vi "capstone2 ver 1.vi"() -> ()   [LabVIEW 2016]
uses:
  <instrlib>/Dynamixel Motor/Public/Motor Operation/Low Level/Baud Setting.ctl
  <vilib>/myRIO/Instrument Drivers/Onboard IO/DIO/typedefs/DIO Reference.ctl
  <vilib>/myRIO/Common/Instrument Driver Framework/Utilities/typedefs/myRIO Generic Hardware Reference.ctl
  <vilib>/myRIO/Common/Instrument Driver Framework/Utilities/typedefs/Hardware Version Enum.ctl
  <vilib>/myRIO/Common/Instrument Driver Framework/Utilities/typedefs/myRIO v1.0 Reference.ctl
  <vilib>/myRIO/Common/Instrument Driver Framework/Utilities/typedefs/Generic FPGA Reference.ctl
  <vilib>/myRIO/Common/Instrument Driver Framework/myRIO v1.0/DIO/typedefs/DIO Channels List.ctl
  <vilib>/myRIO/Common/Instrument Driver Framework/myRIO v1.0/DIO/typedefs/DIO Channels Enum.ctl
  <vilib>/userdefined/High Color/nirio_resource_hc.ctl
  <vilib>/myRIO/Common/Instrument Driver Framework/Utilities/vis/Is FPGA Ref Available.vi
  <vilib>/myRIO/Common/Instrument Driver Framework/myRIO v1.0/DIO/vis/myRIO v1.1 Open DIO.vi
  <vilib>/myRIO/Instrument Drivers/Onboard IO/DIO/vis/Write.vi
  <vilib>/myRIO/Common/Instrument Driver Framework/Utilities/vis/Validate Channels.vi
  <vilib>/myRIO/Common/Instrument Driver Framework/myRIO v1.0/DIO/vis/myRIO v1.0 Reserve DIO.vi
  <vilib>/myRIO/Common/Instrument Driver Framework/myRIO v1.0/UART/vis/myRIO v1.0 Close UART.vi
  <vilib>/myRIO/Common/Instrument Driver Framework/myRIO v1.0/Resource Manager/vis/myRIO v1.0 Reserve Channel List.vi
  <vilib>/myRIO/Common/Instrument Driver Framework/myRIO v1.0/DIO/vis/myRIO v1.0 Build MUX Configuration DIO.vi
  <vilib>/myRIO/Common/Instrument Driver Framework/myRIO v1.0/Resource Manager/vis/myRIO v1.0 Reserve Channel.vi
  <vilib>/myRIO/Common/Instrument Driver Framework/myRIO v1.0/Resource Manager/vis/myRIO v1.0 Unreserve Channel.vi
  <vilib>/myRIO/Common/Instrument Driver Framework/myRIO v1.0/Resource Manager/vis/myRIO v1.0 Create Configuration List.vi
  <vilib>/myRIO/Common/Instrument Driver Framework/myRIO v1.0/Resource Manager/vis/myRIO v1.0 Build Mutex Name.vi
  <vilib>/Utility/VariantDataType/GetNumericInfo.vi
  <vilib>/Utility/error.llb/Error Cluster From Error Code.vi
  <vilib>/myRIO/Common/Instrument Driver Framework/myRIO v1.0/myRIO v1.1 Open.vi
  <vilib>/myRIO/Common/Instrument Driver Framework/Utilities/vis/IO Manager.vi
  <vilib>/myRIO/Common/Instrument Driver Framework/Utilities/vis/Configuration Manager.vi
  <vilib>/myRIO/Common/Instrument Driver Framework/myRIO v1.0/Resource Manager/vis/myRIO v1.0 Configure IO.vi
  <vilib>/myRIO/Common/Instrument Driver Framework/myRIO v1.0/myRIO v1.0 Close.vi
  <vilib>/myRIO/Common/Instrument Driver Framework/myRIO v1.0/DIO/vis/myRIO v1.0 Write DIO.vi
  <vilib>/myRIO/Common/Instrument Driver Framework/Utilities/vis/FPGA Ref Manager.vi
  <vilib>/myRIO/Common/Instrument Driver Framework/myRIO v1.0/myRIO v1.0 Reset FPGA.vi
  <vilib>/myRIO/Common/Instrument Driver Framework/myRIO v1.0/IRQ/vis/myRIO v1.0 IRQ Info FGV.vi
  <vilib>/myRIO/Common/Instrument Driver Framework/myRIO v1.0/IRQ/vis/myRIO v1.0 Timer IRQ Info FGV.vi
  <vilib>/myRIO/Common/Instrument Driver Framework/myRIO v1.0/IRQ/vis/myRIO v1.0 ISR Agent.vi
  <vilib>/myRIO/Express VI/Onboard Devices/LED/LED Express VI.xnode
  <vilib>/myRIO/Instrument Drivers/Onboard IO/DIO/vis/myRIO DIO Open.xnode
  <instrlib>/Dynamixel Motor/Dynamixel Motor.lvlib
  <vilib>/myRIO/Instrument Drivers/Onboard IO/DIO/DIO.lvlib
  <vilib>/myRIO/Instrument Drivers/Utilities/Utilities.lvlib
panel:
  in  "main stop":bool
  out "RT TCP Loop time":u32
  out "motor temp":cluster{"0":sgl, "1":sgl, "2":sgl, "3":sgl}
  out "value":T1
  out "TCP Read data":string
  in  "정지":bool
  out "error out":errorcluster
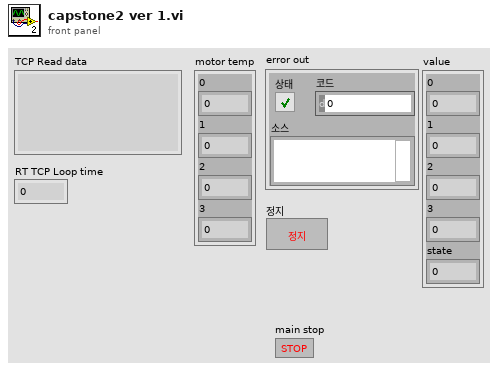
[diagram p1: front panel]
types:
  T1 = cluster{"0":sgl, "1":sgl, "2":sgl, "3":sgl, "state":sgl}
  T2 = typedef "DIO.lvlib/DIO Reference.ctl" = cluster{"myRIO Reference":T3, "DIO Channels List":T7}
  T3 = typedef "myRIO Generic Hardware Reference.ctl" = cluster{"myRIO Model":T4, "myRIO Hardware Reference":T5}
  T4 = typedef "Hardware Version Enum.ctl" = enum16{"Unknown", "myRIO-1900", "myRIO-1950", "roboRIO", "NI ELVIS RIO CM"}
  T5 = typedef "myRIO v1.0 Reference.ctl" = cluster{"Generic FPGA Reference":T6, "Allow multiple opens":bool}
  T6 = typedef "Generic FPGA Reference.ctl" = refnum<k20>
  T7 = typedef "DIO Channels List.ctl" = T8[]
  T8 = typedef "DIO Channels Enum.ctl" = enum16{"Not Connected", "C/DIO0", "C/DIO1", "C/DIO2", "C/DIO3", "C/DIO4", "C/DIO5", "C/DIO6", "C/DIO7", "A/DIO0", "A/DIO1", "A/DIO2", "A/DIO3", "A/DIO4", "A/DIO5", "A/DIO6", "A/DIO7", "A/DIO8", "A/DIO9", "A/DIO10", "A/DIO11", "A/DIO12", "A/DIO13", "A/DIO14", "A/DIO15", "B/DIO0", "B/DIO1", "B/DIO2", "B/DIO3", "B/DIO4", "B/DIO5", "B/DIO6", "B/DIO7", "B/DIO8", "B/DIO9", "B/DIO10", "B/DIO11", "B/DIO12", "B/DIO13", "B/DIO14", "B/DIO15", "LED0", "LED1", "LED2", "LED3", "Button0", "DIO/DIO0", "DIO/DIO1", "DIO/DIO2", "DIO/DIO3", "DIO/DIO4", "DIO/DIO5", "DIO/DIO6", "DIO/DIO7", "DIO/DIO8", "DIO/DIO9", "SPI/CS0", "SPI/CS1", "SPI/CS2", "SPI/CS3", "LED RADIO (Green)", "LED RADIO (Red)", "LED COMM (Green)", "LED COMM (Red)", "LED MODE (Green)", "LED MODE (Red)"}
  T9 = typedef "nirio_resource_hc.ctl" = tag
  T10 = cluster{"0":sgl, "1":sgl, "2":sgl, "3":sgl, "state":i32}
  T11 = typedef "Dynamixel Motor.lvlib/Baud Setting.ctl" = u8
  T12 = enum16{"big-endian, network order", "native, host order", "little-endian"}
  T13 = cluster{"Temperature (C)":u8, "Temperature (C)":u8, "Temperature (C)":u8, "Temperature (C)":u8}
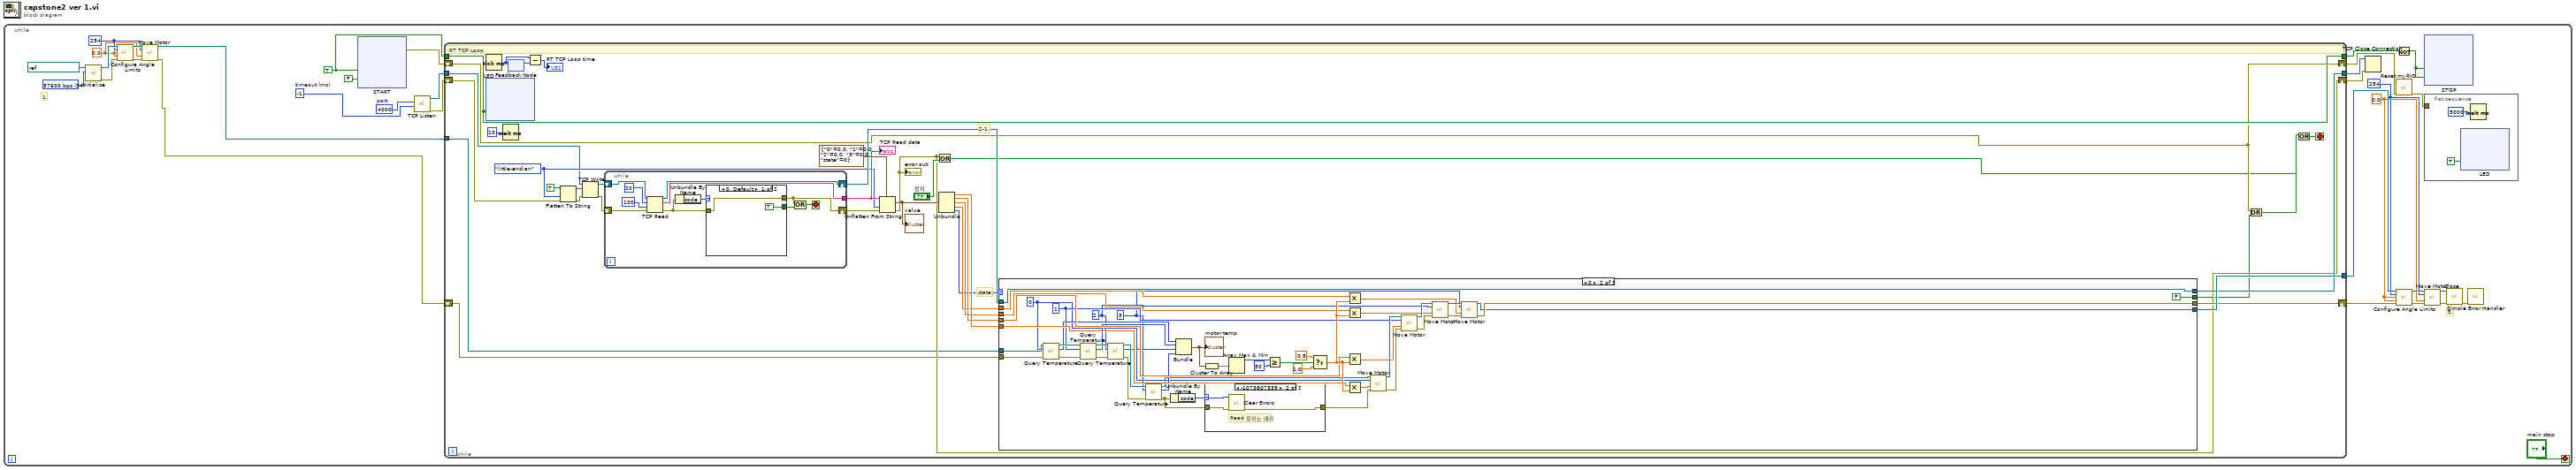
[diagram p0: block diagram]
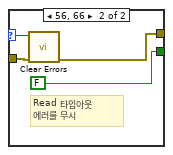
[diagram p2: hidden frame]
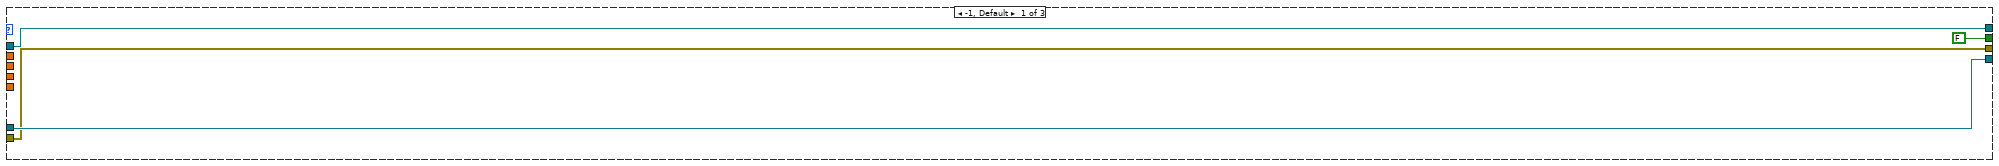
[diagram p3: hidden frame]
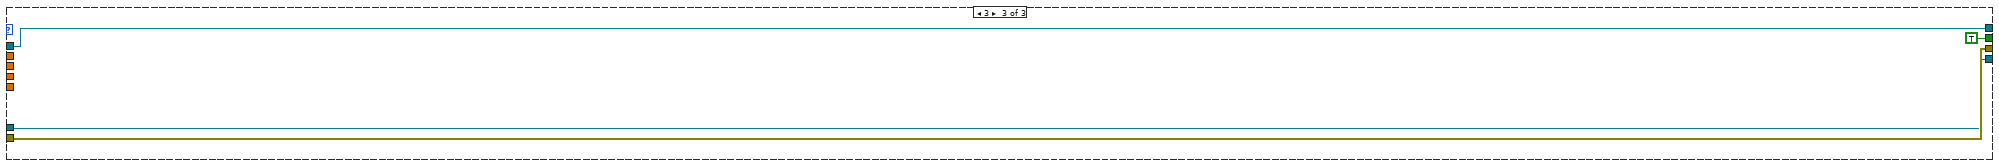
[diagram p5: hidden frame]
diagram:
  n1 = while {
    stop <- "main stop" stop-if-true
    w28 = T11 34 items=["1,000,000 bps"=1, "500,000 bps"=3, "400,000 bps"=4, "250,000 bps"=7, "200,000 bps"=9, "115200 bps"=16, "57600 bps"=34, "19200 bps"=103, "9600 bps"=207] ("Baud rate (57600 bps)")
    w18 = TRUE
    w8 = 0.0 ("Goal Speed (RPM)")
    w9 = u8 254 ("Motor ID (0)")
    w20 = u8 254 ("Motor ID (0)")
    w19 = 0.0 ("Clockwise Angle Limit (0 deg)")
    w32 = u16 4000  # port
    w33 = -1  # timeout (ms)
    # "5."
    # "1."
    n2 = call <instrlib>:"Initialize.vi"("Baud rate (57600 bps)"=w28, "VISA resource name"=refnum<visa-resource-name> "ASRL3::INSTR") -> ("error out"=w24:errorcluster, "VISA resource name out"=w23:refnum<visa-resource-name>)  [unwired: 8 in]
    n3 = call <instrlib>:"Configure Angle Limits.vi"("VISA resource name"=w23, "Motor ID (0)"=w20, "Clockwise Angle Limit (0 deg)"=w19, "Counter-Clockwise Angle Limit (300 deg)"=w19, "error in (no error)"=w24) -> ("VISA resource name out"=w22:refnum<visa-resource-name>, "error out"=w21:errorcluster)  [unwired: 9 in]
    n4 = call <instrlib>:"Move Motor.vi"("VISA resource name"=w22, "Motor ID (0)"=w20, "Goal Speed (RPM)"=w19, "error in (no error)"=w21) -> ("VISA resource name out"=w1:refnum<visa-resource-name>, "error out"=w2:errorcluster)  [unwired: 10 in]
    n5 = xnode "START"("LED0"=w18, "LED3"=FALSE) -> ("error out"=w4:errorcluster)  [unwired: 1 in]
    n6 = call <vilib>:"TCP Listen.vi"("timeout ms (wait forever: -1)"=w33, "port"=w32) -> ("error out"=w29:errorcluster, "connection ID"=w15:refnum<k5>)  [unwired: 5 in, 3 out]
    n7 = while {
      tunnel: w15 -> [w153]
      tunnel: [w158] -> w31
      shift-right: [w149] -> w30
      shift-left: w29 -> [w150]
      shift-right: [w165] -> w13
      shift-left: w2 -> [w164]
      tunnel: w18 -> [w173]
      tunnel: [w173] -> w26
      tunnel: [w166] -> w11
      shift-right: [w144] -> w3
      shift-left: w4 -> [w144]
      tunnel: w1 -> [w146]
      stop <- w147 stop-if-true
      w154 = T12."little-endian" ("byte order (0:big-endian, network order)")
      # "state."
      # "2-1."
      # "RT TCP Loop"
      n8 = Tick Count (ms)() -> (millisecond timer value=w162:u32)
      n9 = xnode "LED"("LED1"=w173) -> ()  [unwired: 1 in, 1 out]
      n10 = Wait (ms)(milliseconds to wait=u32 10 ("대기 시간 (ms)")) -> ()  [unwired: 1 out]
      n11 = feedback #1() -> (w163:u32)  [unwired: 1 in]
      n12 = feedback-in #1(w162) -> ()
      n13 = Subtract(x=w162, y=w163) -> (x-y=→"RT TCP Loop time":u32)
      n14 = Flatten To String(anything=TRUE, byte order (0:big-endian, network order)=w154, error in (no error)=w150) -> (data string=w157:string, error out=w156:errorcluster)  [unwired: 1 in, 1 out]
      n15 = TCP Write(connection ID=w153, data in=w157, error in (no error)=w156) -> (connection ID out=w152:refnum<k5>, error out=w151:errorcluster)  [unwired: 1 in, 1 out]
      n16 = while {
        tunnel: [w186] -> w175
        shift-right: [w185] -> w159
        shift-left: w152 -> [w184]
        shift-right: [w180] -> w174
        shift-left: w151 -> [w183]
        stop <- w178 stop-if-true
        n17 = TCP Read(connection ID=w184, bytes to read=20 ("읽을 바이트"), error in (no error)=w183, 9:100 ("타임아웃 ms (25000)")) -> (connection ID out=w185:refnum<k5>, data out=w186:string, error out=w181:errorcluster)  [unwired: 1 in]
        n18 = Unbundle By Name(w181) -> ("code"=w182:i32)
        n19 = case shown="0, Default" w182 {
          selector: w182 -> [_ w193]
          tunnel: [w190 w192] -> w180
          tunnel: w181 -> [w190 w194]
          tunnel: [TRUE FALSE] -> w179
          frame 0, Default {
          }
          frame 56, 66 {
            # "Read 타임아웃\n에러를 무시"
            n20 = call <vilib>:"Clear Errors.vi"("error in (no error)"=w194, "specific error code to clear (0: all)"=w193) -> ("error out"=w192:errorcluster)  [unwired: 4 in, 1 out]
          }
        }
        n21 = Or(x=w180, y=w179) -> (x .or. y?=w178:bool)
      }
      "TCP Read data" <- w175
      n22 = Unflatten From String(type=T10 {"0"=0.0, "1"=0.0, "2"=0.0, "3"=0.0, "state"=0}, binary string=w175, byte order (0:big-endian, network order)=w154, error in (no error)=w174) -> (value=w172:T10, error out=w149:errorcluster)  [unwired: 1 in, 1 out]
      "error out" <- w149
      "value" <- w172
      n23 = Or(x=w149, y="정지") -> (x .or. y?=w143:bool)
      n24 = Unbundle(w172) -> ("0"=w171:sgl, "1"=w169:sgl, "2"=w170:sgl, "3"=w168:sgl, "state"=w167:i32)
      n25 = case shown="0" w167 {
        tunnel: w171 -> [_ w228 _]
        tunnel: w169 -> [_ w227 _]
        tunnel: w170 -> [_ w226 _]
        tunnel: w168 -> [_ w225 _]
        tunnel: [w198 w210 w249] -> w166
        tunnel: [w197 w211 w250] -> w165
        tunnel: w164 -> [w197 w208 w250]
        tunnel: w146 -> [w198 w201 w249]
        tunnel: w159 -> [w196 w200 w252]
        tunnel: [w196 w200 w252] -> w158
        tunnel: [FALSE FALSE TRUE] -> w145
        frame -1, Default {
        }
        frame 0 {
          w212 = 3
          w213 = 2
          w214 = 1
          w209 = 0
          n26 = call <instrlib>:"Query Temperature.vi"("error in"=w208, "Motor ID (0)"=w209, "VISA resource name"=w201) -> ("error out"=w235:errorcluster, "Temperature (C)"=w224:u8, "VISA resource name out"=w238:refnum<visa-resource-name>)  [unwired: 6 in]
          n27 = call <instrlib>:"Query Temperature.vi"("error in"=w235, "Motor ID (0)"=w214, "VISA resource name"=w238) -> ("error out"=w234:errorcluster, "Temperature (C)"=w223:u8, "VISA resource name out"=w237:refnum<visa-resource-name>)  [unwired: 6 in]
          n28 = call <instrlib>:"Query Temperature.vi"("error in"=w234, "Motor ID (0)"=w213, "VISA resource name"=w237) -> ("error out"=w233:errorcluster, "Temperature (C)"=w222:u8, "VISA resource name out"=w236:refnum<visa-resource-name>)  [unwired: 6 in]
          n29 = call <instrlib>:"Query Temperature.vi"("error in"=w233, "Motor ID (0)"=w212, "VISA resource name"=w236) -> ("error out"=w215:errorcluster, "Temperature (C)"=w221:u8, "VISA resource name out"=w207:refnum<visa-resource-name>)  [unwired: 6 in]
          n30 = Unbundle By Name(w215) -> ("code"=w216:i32)
          n31 = Bundle("Temperature (C)"=w224, "Temperature (C)"=w223, "Temperature (C)"=w222, "Temperature (C)"=w221) -> (w218:T13)  [unwired: 1 in]
          "motor temp" <- w218
          n32 = Cluster To Array(cluster=w218) -> (array=w220:u8[])
          n33 = case shown="-1073807339" w216 {
            selector: w216 -> [_ w247]
            tunnel: [w245 w246] -> w206
            tunnel: w215 -> [w245 w248]
            frame 0, Default {
            }
            frame -1073807339 {
              # "Read 못하는 에러"
              n34 = call <vilib>:"Clear Errors.vi"("error in (no error)"=w248, "specific error code to clear (0: all)"=w247) -> ("error out"=w246:errorcluster)  [unwired: 4 in, 1 out]
            }
          }
          n35 = Array Max & Min(array=w220) -> (max value=w219:u8)  [unwired: 3 out]
          n36 = Greater Or Equal?(x=w219, y=50) -> (x >= y?=w217:bool)
          n37 = Select(t=0.5, s=w217, f=1.0) -> (s? t:f=w229:dbl)
          n38 = Multiply(x=w225, y=w229) -> (x*y=w202:dbl)
          n39 = Multiply(x=w226, y=w229) -> (x*y=w203:dbl)
          n40 = Multiply(x=w227, y=w229) -> (x*y=w204:dbl)
          n41 = Multiply(x=w228, y=w229) -> (x*y=w205:dbl)
          n42 = call <instrlib>:"Move Motor.vi"("VISA resource name"=w207, "Motor ID (0)"=w209, "Goal Speed (RPM)"=w205, "error in (no error)"=w206) -> ("VISA resource name out"=w239:refnum<visa-resource-name>, "error out"=w240:errorcluster)  [unwired: 10 in]
          n43 = call <instrlib>:"Move Motor.vi"("VISA resource name"=w239, "Motor ID (0)"=w214, "Goal Speed (RPM)"=w204, "error in (no error)"=w240) -> ("VISA resource name out"=w241:refnum<visa-resource-name>, "error out"=w243:errorcluster)  [unwired: 10 in]
          n44 = call <instrlib>:"Move Motor.vi"("VISA resource name"=w241, "Motor ID (0)"=w213, "Goal Speed (RPM)"=w203, "error in (no error)"=w243) -> ("VISA resource name out"=w242:refnum<visa-resource-name>, "error out"=w244:errorcluster)  [unwired: 10 in]
          n45 = call <instrlib>:"Move Motor.vi"("VISA resource name"=w242, "Motor ID (0)"=w212, "Goal Speed (RPM)"=w202, "error in (no error)"=w244) -> ("VISA resource name out"=w210:refnum<visa-resource-name>, "error out"=w211:errorcluster)  [unwired: 10 in]
        }
        frame 3 {
        }
      }
      n46 = Or(x=w144, y=w145) -> (x .or. y?=w148:bool)
      n47 = Or(x=w148, y=w143) -> (x .or. y?=w147:bool)
    }
    n48 = TCP Close Connection(connection ID=w31, error in (no error)=w30) -> ()  [unwired: 3 out]
    n49 = Not(x=w26) -> (.not. x?=w25:bool)
    n50 = call <vilib>:"Reset myRIO.vi"("error in (no error)"=w3) -> ("error out"=w7:errorcluster)  [unwired: 10 in]
    n51 = call <instrlib>:"Configure Angle Limits.vi"("VISA resource name"=w11, "Motor ID (0)"=w9, "Clockwise Angle Limit (0 deg)"=w8, "Counter-Clockwise Angle Limit (300 deg)"=w8, "error in (no error)"=w13) -> ("VISA resource name out"=w10:refnum<visa-resource-name>, "error out"=w12:errorcluster)  [unwired: 9 in]
    n52 = xnode "STOP"("LED0"=w25, "LED1"=w25) -> ()  [unwired: 1 in, 1 out]
    n53 = flat-sequence {
      tunnel: w7 -> [_]
      frame #0 {
        n54 = xnode "LED"("LED3"=TRUE) -> ()  [unwired: 1 in, 1 out]
        n55 = Wait (ms)(milliseconds to wait=5000) -> ()  [unwired: 1 out]
      }
    }
    n56 = call <instrlib>:"Move Motor.vi"("VISA resource name"=w10, "Motor ID (0)"=w9, "Goal Speed (RPM)"=w8, "error in (no error)"=w12) -> ("VISA resource name out"=w17:refnum<visa-resource-name>, "error out"=w16:errorcluster)  [unwired: 10 in]
    n57 = call <instrlib>:"Close.vi"("error in (no error)"=w16, "VISA resource name"=w17) -> ("error out"=w14:errorcluster)  [unwired: 9 in]
    n58 = call <vilib>:"Simple Error Handler.vi"("error in (no error)"=w14) -> ()  [unwired: 4 in, 5 out]
  }
